vi "GFITS_ParseDataType.vi"(10 "string type":string) -> (2 "numeric type":i32)   [LabVIEW 2016]
uses:
  GFITS_datatypesctl.ctl
panel:
  in  "Types":T1={"TBIT"=1, "TBYTE"=11, "TSTRING"=16, "TSHORT"=21, "TLONG"=41, "TFLOAT"=42, "TDOUBLE"=82, "TCOMPLEX"=83, "TDBLCOMPLEX"=163, "TUINT"=30, "TUSHORT"=20, "TULONG"=40, "TINT"=31, "TSBYTE"=12, "TLONGLONG"=81, "TLOGICAL"=14}
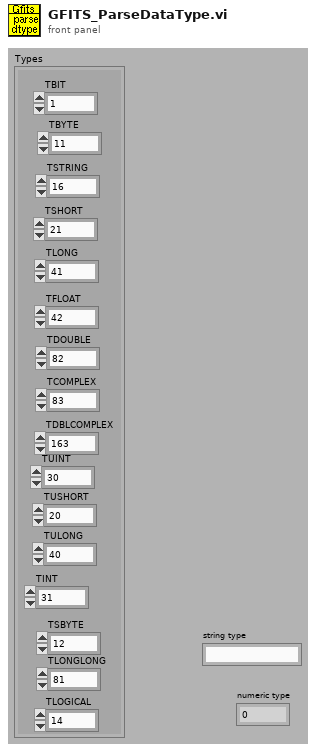
[diagram p1: front panel]
types:
  T1 = typedef "GFITS_datatypesctl.ctl" = cluster{"TBIT":i32, "TBYTE":i32, "TSTRING":i32, "TSHORT":i32, "TLONG":i32, "TFLOAT":i32, "TDOUBLE":i32, "TCOMPLEX":i32, "TDBLCOMPLEX":i32, "TUINT":i32, "TUSHORT":i32, "TULONG":i32, "TINT":i32, "TSBYTE":i32, "TLONGLONG":i32, "TLOGICAL":i32}
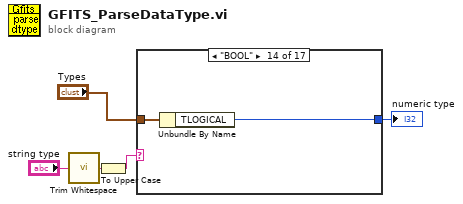
[diagram p0: block diagram]
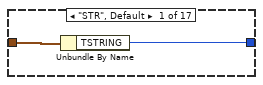
[diagram p2: hidden frame]
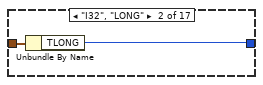
[diagram p3: hidden frame]
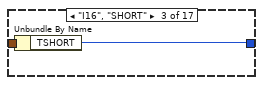
[diagram p4: hidden frame]
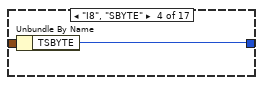
[diagram p5: hidden frame]
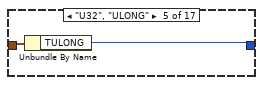
[diagram p6: hidden frame]
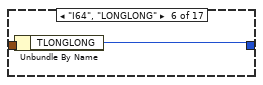
[diagram p7: hidden frame]
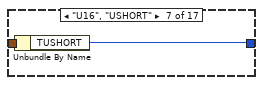
[diagram p8: hidden frame]
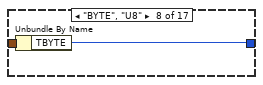
[diagram p9: hidden frame]
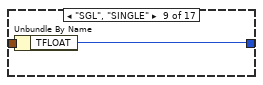
[diagram p10: hidden frame]
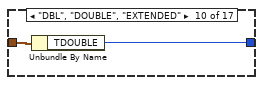
[diagram p11: hidden frame]
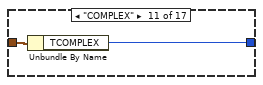
[diagram p12: hidden frame]
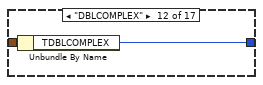
[diagram p13: hidden frame]
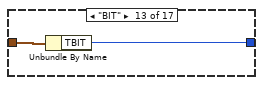
[diagram p14: hidden frame]
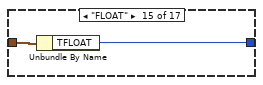
[diagram p15: hidden frame]
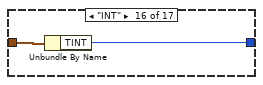
[diagram p16: hidden frame]
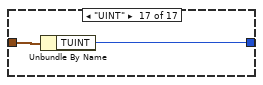
[diagram p17: hidden frame]
diagram:
  n1 = call <vilib>:"Trim Whitespace.vi"("string"="string type") -> ("trimmed string"=w2:string)  [unwired: 1 in]
  n2 = To Upper Case(1:w2) -> (0:w1:string)
  n3 = case shown="\"BOOL\"" w1 {
    tunnel: [w7 w9 w11 w13 w15 w17 w19 w21 w23 w25 w27 w29 w31 w33 w35 w37 w39] -> w3
    tunnel: "Types" -> [w6 w8 w10 w12 w14 w16 w18 w20 w22 w24 w26 w28 w30 w32 w34 w36 w38]
    frame "STR", Default {
      n4 = Unbundle By Name(w6) -> ("TSTRING"=w7:i32)
    }
    frame "I32", "LONG" {
      n5 = Unbundle By Name(w8) -> ("TLONG"=w9:i32)
    }
    frame "I16", "SHORT" {
      n6 = Unbundle By Name(w10) -> ("TSHORT"=w11:i32)
    }
    frame "I8", "SBYTE" {
      n7 = Unbundle By Name(w12) -> ("TSBYTE"=w13:i32)
    }
    frame "U32", "ULONG" {
      n8 = Unbundle By Name(w14) -> ("TULONG"=w15:i32)
    }
    frame "I64", "LONGLONG" {
      n9 = Unbundle By Name(w16) -> ("TLONGLONG"=w17:i32)
    }
    frame "U16", "USHORT" {
      n10 = Unbundle By Name(w18) -> ("TUSHORT"=w19:i32)
    }
    frame "BYTE", "U8" {
      n11 = Unbundle By Name(w20) -> ("TBYTE"=w21:i32)
    }
    frame "SGL", "SINGLE" {
      n12 = Unbundle By Name(w22) -> ("TFLOAT"=w23:i32)
    }
    frame "DBL", "DOUBLE", "EXTENDED" {
      n13 = Unbundle By Name(w24) -> ("TDOUBLE"=w25:i32)
    }
    frame "COMPLEX" {
      n14 = Unbundle By Name(w26) -> ("TCOMPLEX"=w27:i32)
    }
    frame "DBLCOMPLEX" {
      n15 = Unbundle By Name(w28) -> ("TDBLCOMPLEX"=w29:i32)
    }
    frame "BIT" {
      n16 = Unbundle By Name(w30) -> ("TBIT"=w31:i32)
    }
    frame "BOOL" {
      n17 = Unbundle By Name(w32) -> ("TLOGICAL"=w33:i32)
    }
    frame "FLOAT" {
      n18 = Unbundle By Name(w34) -> ("TFLOAT"=w35:i32)
    }
    frame "INT" {
      n19 = Unbundle By Name(w36) -> ("TINT"=w37:i32)
    }
    frame "UINT" {
      n20 = Unbundle By Name(w38) -> ("TUINT"=w39:i32)
    }
  }
  "numeric type" <- w3
